vi "BEGIN.vi"(7 "Savepoint name":string, 8 "error in (no error)":errorcluster, 11 "PQ Connection in":refnum<class "PQ Connection.lvclass">) -> (0 "error out":errorcluster, 3 "PQ Connection out":refnum<class "PQ Connection.lvclass">)   [LabVIEW 2015, in "PQ Connection.lvclass"]
doc: "Start a transaction using \"BEGIN\". \n\nIf an optional Savepoint name is provided then a SAVEPOINT is created instead. Savepoints can be nested."
uses:
  PQ Connection.lvclass
  Result/PQ Result.lvclass/PQ Result.ctl
  Result/Clear.vi
  Execute (Return first result with rows).vi
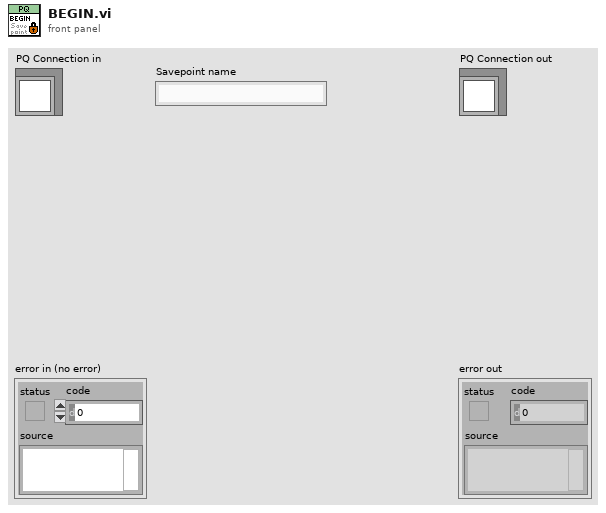
[diagram p1: front panel]
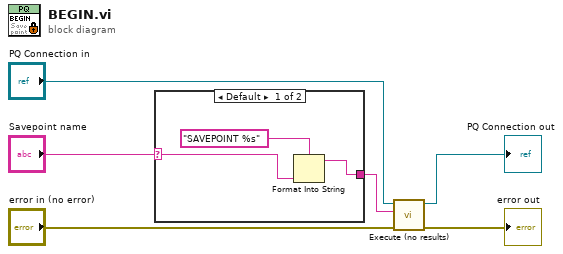
[diagram p0: block diagram]
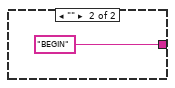
[diagram p2: hidden frame]
diagram:
  n1 = case shown="Default" "Savepoint name" {
    selector: "Savepoint name" -> [w9 _]
    tunnel: [w7 "BEGIN"] -> w1
    frame Default {
      n2 = Format Into String(format string="SAVEPOINT %s", w9) -> (resulting string=w7:string)  [unwired: 2 in, 1 out]
    }
    frame "" {
    }
  }
  n3 = call "Execute (no results).vi"("error in (no error)"="error in (no error)", "SQL"=w1, "PQ Connection in"="PQ Connection in") -> ("error out"=→"error out":errorcluster, "PQ Connection out"=→"PQ Connection out":refnum<class "PQ Connection.lvclass">)  [unwired: 7 in]
